vi "Launch Nested Actors.vi"(8 "error in (no error)":errorcluster, 10 "Selection UI Subpanel Ref":refnum<vi>, 11 "Pane Relief Main UI in":refnum<class "Pane Relief Main UI.lvclass">) -> (0 "error out":errorcluster, 3 "Pane Relief Main UI out":refnum<class "Pane Relief Main UI.lvclass">)   [LabVIEW 2018, in "Pane Relief Main UI.lvlib" / "Pane Relief Main UI.lvclass"]
uses:
  <resource>/dialog/QuickDrop/plugins/PaneRelief/Classes/Pane Relief Main UI/Pane Relief Main UI/Pane Relief Main UI.lvclass
  C:/Program Files (x86)/National Instruments/LabVIEW 2018/vi.lib/MGI/Panel Manager/Panel Actor/Panel Actor/Panel Actor.lvclass
  <resource>/dialog/QuickDrop/plugins/PaneRelief/Classes/Splitter Settings UI/Splitter Settings UI/Splitter Settings UI.lvclass
  <resource>/dialog/QuickDrop/plugins/PaneRelief/Classes/Pane Settings UI/Pane Settings UI/Pane Settings UI.lvclass
  <resource>/dialog/QuickDrop/plugins/PaneRelief/Classes/Panel Object Actions UI/Panel Object Actions UI/Panel Object Actions UI.lvclass
  <resource>/dialog/QuickDrop/plugins/PaneRelief/Classes/Instructions UI/Instructions UI/Instructions UI.lvclass
  <resource>/dialog/QuickDrop/plugins/PaneRelief/Classes/Pane Relief Main UI/Pane Relief Main UI/Pane Relief Main UI.lvclass/Pane Relief Main UI.ctl
  <vilib>/MGI/Panel Manager/Panel/Panel/Subpanel/Subpanel.lvclass
  C:/Program Files (x86)/National Instruments/LabVIEW 2018/vi.lib/MGI/Panel Manager/Panel/Panel/Panel.lvclass
  <vilib>/MGI/Panel Manager/Panel/Panel/Subpanel/Subpanel.vi
  <vilib>/MGI/Panel Manager/Panel Actor/Panel Actor/Panel Actor.lvclass
  <vilib>/MGI/Panel Manager/Panel/Panel.lvlib
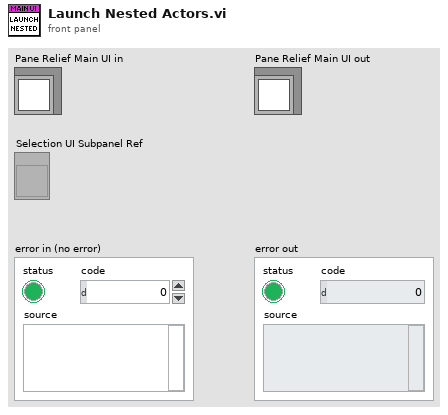
[diagram p1: front panel]
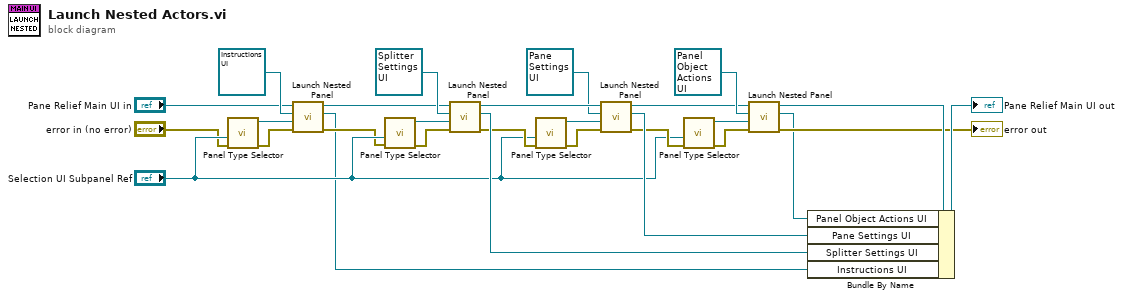
[diagram p0: block diagram]
diagram:
  n1 = call-poly <vilib>:"Panel Type Selector.vi"("Error In"="error in (no error)", "Sub Panel"="Selection UI Subpanel Ref") -> ("Error Out"=w8:errorcluster, "Subpanel Out"=w9:refnum<class "Subpanel.lvclass">)  [unwired: 8 in]
  n2 = call <vilib>:"Launch Nested Panel.vi"("error in (no error)"=w8, "Panel"=w9, "Nested Panel Actor"=refnum<class "Instructions UI.lvclass"> refnum ("Instructions UI.lvlib:Instructions UI.lvclass"), "Panel Actor in"="Pane Relief Main UI in") -> ("error out"=w4:errorcluster, "Nested Actor's Enqueuer"=w1:refnum<class "Message Enqueuer.lvclass">, "Panel Actor out"=w2:refnum<class "Pane Relief Main UI.lvclass">)  [unwired: 4 in, 1 out]
  n3 = call-poly <vilib>:"Panel Type Selector.vi"("Error In"=w4, "Sub Panel"="Selection UI Subpanel Ref") -> ("Error Out"=w19:errorcluster, "Subpanel Out"=w18:refnum<class "Subpanel.lvclass">)  [unwired: 8 in]
  n4 = call <vilib>:"Launch Nested Panel.vi"("error in (no error)"=w19, "Panel"=w18, "Nested Panel Actor"=refnum<class "Splitter Settings UI.lvclass"> refnum ("Splitter Settings UI.lvlib:Splitter Settings UI.lvclass"), "Panel Actor in"=w2) -> ("error out"=w25:errorcluster, "Nested Actor's Enqueuer"=w27:refnum<class "Message Enqueuer.lvclass">, "Panel Actor out"=w24:refnum<class "Pane Relief Main UI.lvclass">)  [unwired: 4 in, 1 out]
  n5 = call-poly <vilib>:"Panel Type Selector.vi"("Error In"=w25, "Sub Panel"="Selection UI Subpanel Ref") -> ("Error Out"=w22:errorcluster, "Subpanel Out"=w23:refnum<class "Subpanel.lvclass">)  [unwired: 8 in]
  n6 = call <vilib>:"Launch Nested Panel.vi"("error in (no error)"=w22, "Panel"=w23, "Nested Panel Actor"=refnum<class "Pane Settings UI.lvclass"> refnum ("Pane Settings UI.lvlib:Pane Settings UI.lvclass"), "Panel Actor in"=w24) -> ("error out"=w14:errorcluster, "Nested Actor's Enqueuer"=w26:refnum<class "Message Enqueuer.lvclass">, "Panel Actor out"=w13:refnum<class "Pane Relief Main UI.lvclass">)  [unwired: 4 in, 1 out]
  n7 = call-poly <vilib>:"Panel Type Selector.vi"("Error In"=w14, "Sub Panel"="Selection UI Subpanel Ref") -> ("Error Out"=w16:errorcluster, "Subpanel Out"=w15:refnum<class "Subpanel.lvclass">)  [unwired: 8 in]
  n8 = call <vilib>:"Launch Nested Panel.vi"("error in (no error)"=w16, "Panel"=w15, "Nested Panel Actor"=refnum<class "Panel Object Actions UI.lvclass"> refnum ("Panel Object Actions UI.lvlib:Panel Object Actions UI.lvclass"), "Panel Actor in"=w13) -> ("error out"=→"error out":errorcluster, "Nested Actor's Enqueuer"=w10:refnum<class "Message Enqueuer.lvclass">, "Panel Actor out"=w12:refnum<class "Pane Relief Main UI.lvclass">)  [unwired: 4 in, 1 out]
  n9 = Bundle By Name(cluster=w12, "Panel Object Actions UI"=w10, "Pane Settings UI"=w26, "Splitter Settings UI"=w27, "Instructions UI"=w1) -> (→"Pane Relief Main UI out":refnum<class "Pane Relief Main UI.lvclass">)
